vi "Display Console - Input Messages.vi"(8 "error in (no error)":errorcluster, 11 "View Model":T1) -> (0 "error out":errorcluster, 3 "View Model":T1)   [LabVIEW 2017]
doc: "Provides Input a list of messages from external text file.\n[Covers: UM1]"
uses:
  View Model/Controls/View Model.ctl
  Error Handler/Controls/Error Model.ctl
  Error Handler/Controls/Error Data.ctl
  Error Handler/Controls/Error Type.ctl
  View Model/Controls/Shared Model.ctl
  Configuration/Controls/Config Model.ctl
  Configuration/Controls/Config CMD.ctl
  Configuration/Controls/Config Data.ctl
  ATM Controller/Controls/Controller Model.ctl
  ATM Controller/Controls/Controller Overhead.ctl
  ATM Controller/Controls/Controller States.ctl
  ATM Controller/Controls/Controller Message Data.ctl
  ATM Controller/Controls/Controller CMD.ctl
  User Console View/Controls/User Console - Transaction Enum.ctl
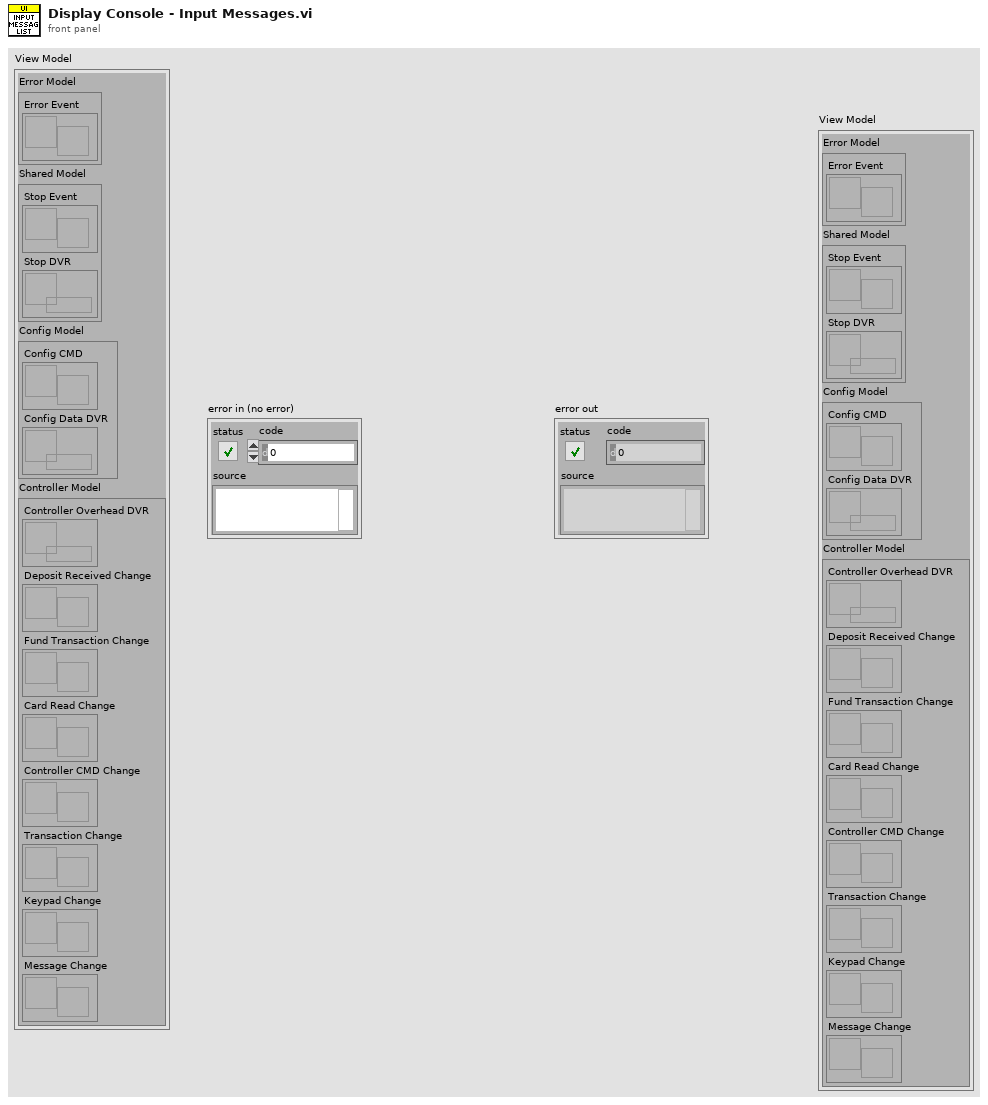
[diagram p1: front panel]
types:
  T1 = typedef "View Model.ctl" = cluster{"Error Model":T2, "Shared Model":T3, "Config Model":T4, "Controller Model":T5}
  T2 = typedef "Error Model.ctl" = cluster{"Error Event":refnum<user-event>}
  T3 = typedef "Shared Model.ctl" = cluster{"Stop Event":refnum<user-event>, "Stop DVR":refnum<data-value>}
  T4 = typedef "Config Model.ctl" = cluster{"Config CMD":refnum<user-event>, "Config Data DVR":refnum<data-value>}
  T5 = typedef "Controller Model.ctl" = cluster{"Controller Overhead DVR":refnum<data-value>, "Deposit Received Change":refnum<user-event>, "Fund Transaction Change":refnum<user-event>, "Card Read Change":refnum<user-event>, "Controller CMD Change":refnum<user-event>, "Transaction Change":refnum<user-event>, "Keypad Change":refnum<user-event>, "Message Change":refnum<user-event>}
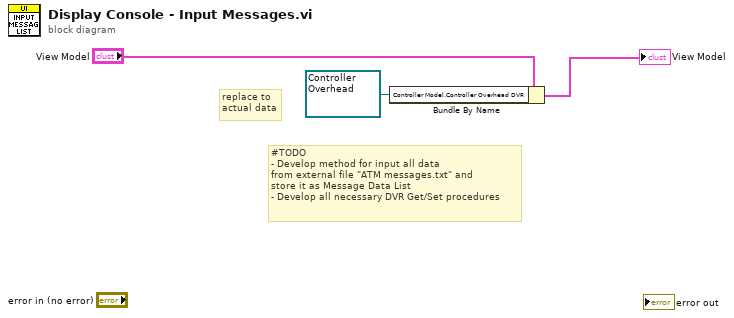
[diagram p0: block diagram]
diagram:
  # "replace to\nactual data"
  # "#TODO\n- Develop method for input all data\nfrom external file \"ATM messages.txt\" and\nstore it as Message Data List\n- Develop all necessary DVR Get/Set procedures"
  n1 = Bundle By Name(cluster="View Model", "Controller Model.Controller Overhead DVR"=refnum<data-value> refnum) -> (→"View Model":T1)
